vi "WriteData.vi"(8 "Error In":errorcluster, 10 "Data":string, 11 "reference in":refnum<class "CompressedEncryptedFileDataSource.lvclass">) -> (0 "Error Out":errorcluster, 3 "reference out":refnum<class "CompressedEncryptedFileDataSource.lvclass">)   [LabVIEW 2020, in "CompressedEncryptedFileDataSource.lvclass"]
uses:
  CompressedEncryptedFileDataSource.lvclass
  EncryptedFileDataSource_class/EncryptedFileDataSource.lvclass
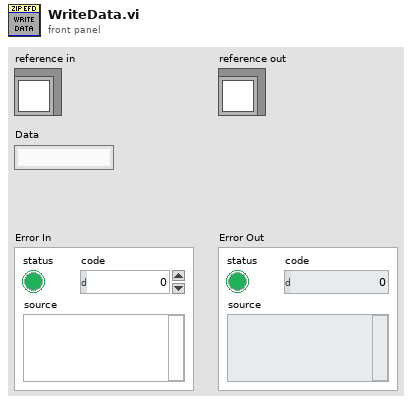
[diagram p1: front panel]
types:
  T1 = typedef "CompressedEncryptedFileDataSource.lvclass/ObjectAttributes.ctl" = cluster{"CompressionType":T2}
  T2 = typedef "CompressedEncryptedFileDataSource.lvclass/EncryptionType.ctl" = enum16{"Type 1", "Type 2"}
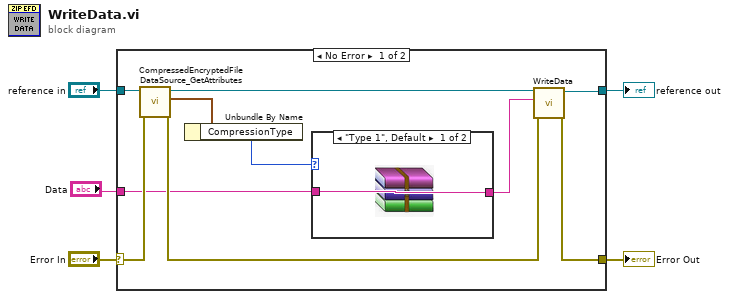
[diagram p0: block diagram]
diagram:
  n1 = case shown="No Error" "Error In" {
    selector: "Error In" -> [w15 w19]
    tunnel: [w9 w19] -> w4
    tunnel: [w11 w18] -> w2
    tunnel: "reference in" -> [w13 w18]
    tunnel: "Data" -> [w7 _]
    frame No Error {
      n2 = call "CompressedEncryptedFileDataSource_GetAttributes.vi"("error in (no error)"=w15, "reference in"=w13) -> ("error out"=w10:errorcluster, "Data"=w14:T1, "reference out"=w12:refnum<class "CompressedEncryptedFileDataSource.lvclass">)  [unwired: 6 in, 1 out]
      n3 = Unbundle By Name(w14) -> ("CompressionType"=w8:T2)
      n4 = case shown="\"Type 1\", Default" w8 {
        tunnel: w7 -> [w16 w17]
        tunnel: [w16 w17] -> w6
        frame "Type 1", Default {
        }
        frame "Type 2" {
        }
      }
      n5 = call-parent "WriteData.vi"("Error In"=w10, "Data"=w6, "reference in"=w12) -> ("Error Out"=w9:errorcluster, "reference in"=w11:refnum<class "CompressedEncryptedFileDataSource.lvclass">)  [unwired: 7 in]
    }
    frame Error {
    }
  }
  "Error Out" <- w4
  "reference out" <- w2
